vi "Configure SAV.vi"(8 "error in (no error)":errorcluster, 10 "decimal":i16=1 min=1 max=99 step=1, 11 "VISA resource name":refnum<visa-resource-name>) -> (0 "error out":errorcluster, 3 "VISA resource name out":refnum<visa-resource-name>)   [LabVIEW 2025, in "Chroma 19052.lvlib"]
uses:
  <instrlib>/Chroma 19052/Chroma 19052.lvlib
panel:
  # "*SAV"
  # "Save currente state"
  # "(See note inside)"
  # "1...99"
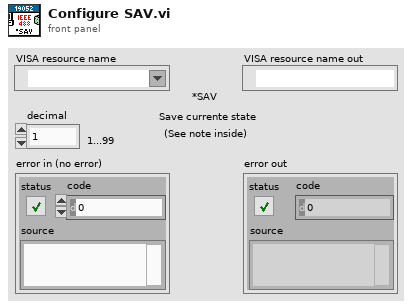
[diagram p1: front panel]
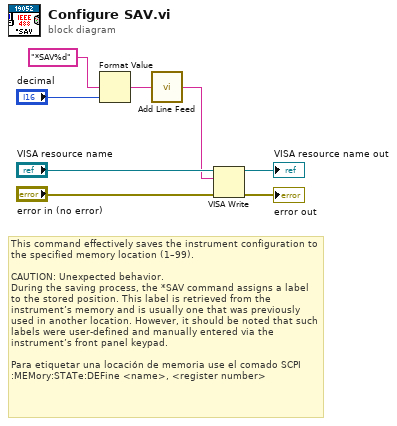
[diagram p0: block diagram]
diagram:
  # "This command effectively saves the instrument configuration to the specified memory location (1–99).\n\nCAUTION: Unexpected behavior.\nDuring the saving process, the *SAV command assigns a label to the stored position. This label is retrieved from the instrument’s memory and is usually one that was previously used in another location. However, it should be noted that such labels were user-defined and manually entered via the instrument’s front panel keypad.\n\nPara etiquetar una locación de memoria use el comado SCPI :MEMory:STATe:DEFine <name>, <register number>"
  n1 = Format Value(format string="*SAV%d", value (0)="decimal") -> (output string=w3:string)  [unwired: 1 in]
  n2 = call <instrlib>:"Add Line Feed.vi"("Command string"=w3) -> ("Concatenated string"=w1:string)  [unwired: 4 in]
  n3 = VISA Write(VISA resource name="VISA resource name", write buffer=w1, error in (no error)="error in (no error)") -> (VISA resource name out=→"VISA resource name out":refnum<visa-resource-name>, error out=→"error out":errorcluster)  [unwired: 1 out]
